vi "MEMR.vi"(11 "Expt State":T6) -> ()   [LabVIEW 2020]
uses:
  CFTS Main Panel SubVIs/CFTS-Experiment State.ctl
  Typedefs/MEMR-Sequence Step.ctl
panel:
  in  "Run":i32
  in  "Number":i32
  in  "ID":string
  out "exit signal":bool
  in  "Sampling rate (Hz)":dbl
  in  "Save raw data?":bool
  in  "Analysis":T1
  in  "Repeats":i32
  in  "Timing":T2
  in  "Sequence":T3
  in  "Elicitor":T4
  in  "Probe":T5
  out "Cal files":string
  out "show cal names":bool
  in  "file pattern":path
  in  "Start":bool
  in  "Stop":bool
  out "running":bool
  out "analysis":errorcluster
  out "finished":errorcluster
  out "restore defaults":bool
  out "ProgressBar":u8(slide) caption="Slide" scale=0.0..28.0
  out "FreqGraph":cluster{dbl[], dbl[]}(graph)
  out "IOGraph":cluster{dbl[], dbl[]}[](graph)
  out "TimeGraph":dbl[][](graph)
  out "GainSpectra":cluster{dbl[], dbl[]}[](graph)
  # "Probe"
  # "Elicitor"
  # "Timing"
  # "Analysis"
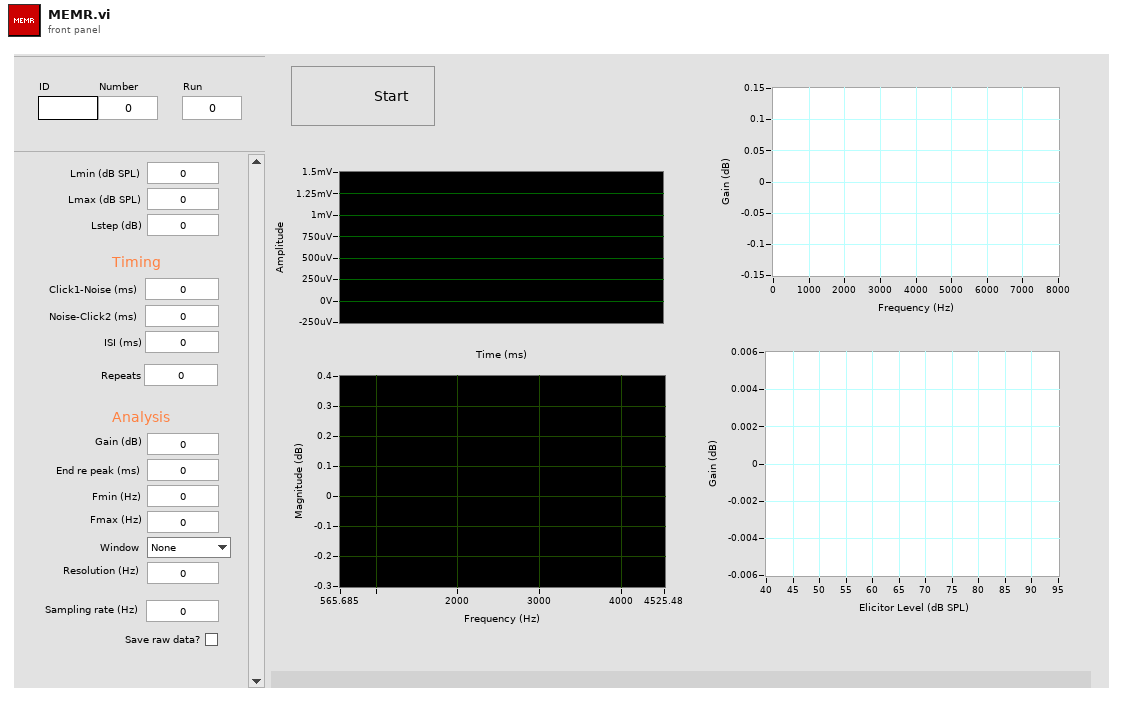
[diagram p1: front panel]
types:
  T1 = cluster{"T(ms) re peak":dbl, "Fmin (Hz)":dbl, "Fmax (Hz)":dbl, "Window":enum16{"None", "Hanning", "Hamming"}, "Gain (dB)":dbl, "Resol (Hz)":dbl}
  T2 = cluster{"Click1-Noise (ms)":dbl, "Noise-Click2 (ms)":dbl, "ISI (ms)":dbl}
  T3 = cluster{"Lmin (dB SPL)":dbl, "Lmax (dB SPL)":dbl, "Lstep (dB)":dbl}
  T4 = cluster{"Duration (ms)":dbl, "Ramp (ms)":dbl, "Transducer":enum16{"Insert", "TDH-39", "HD300", "ER-10X"}}
  T5 = cluster{"Ear":enum16{"Right", "Left"}, "Stimulus":enum16{"Click", "Chirp"}, "Duration (us)":dbl, "Level (dB pSPL)":dbl}
  T6 = typedef "CFTS-Experiment State.ctl" = cluster{"Experimenter":string, "Number":u32, "Right":string, "Left":string, "Data Folder":path, "State File":path, "Version Info":string, "End Exposure Time":dbl, "Exposure Duration":string, "Run #":cluster{"CAP":i16, "ABR":i16, "DP":i16, "VsEP":i16, "MeasSeq":i16, "SubSeq":i16, "SFOAE":i16}}
  T7 = typedef "MEMR-IPC.ctl" = cluster{"SGDA":refnum<queue>, "AnalysisStart":refnum<queue>, "AnalysisUpdate":refnum<queue>}
  T8 = cluster{"Run":refnum<vi>, "ProgressBar":refnum<vi>, "IOGraph":refnum<vi>, "TimeGraph":refnum<vi>, "FreqGraph":refnum<vi>, "GainSpectra":refnum<vi>}
  T9 = typedef "MEMR-Params.ctl" = cluster{"Probe":T10, "Elicitor":T11, "Sequence":T13, "Analysis":T14, "Repeats":i32, "Timing":T15, "Save raw":bool, "Fs (Hz)":dbl}
  T10 = typedef "MEMR-Probe.ctl" = cluster{"Ear":enum16{"Right", "Left"}, "Stimulus":enum16{"Click", "Chirp"}, "Duration (us)":dbl, "Level":dbl}
  T11 = typedef "MEMR-Elicitor.ctl" = cluster{"Duration (ms)":dbl, "Ramp (ms)":dbl, "Transducer":T12}
  T12 = typedef "HSTS-Transducer.ctl" = enum16{"Insert", "TDH-39", "HD300", "ER-10X"}
  T13 = typedef "MEMR-Sequence.ctl" = cluster{"Start":dbl, "Stop":dbl, "Step":dbl}
  T14 = typedef "MEMR-Analysis.ctl" = cluster{"T(ms) re peak":dbl, "Fmin (Hz)":dbl, "Fmax (Hz)":dbl, "Window":enum16{"None", "Hanning", "Hamming"}, "Gain (dB)":dbl, "Resol (Hz)":dbl}
  T15 = typedef "MEMR-Timing.ctl" = cluster{"Click1-Noise (ms)":dbl, "Noise-Click2 (ms)":dbl, "ISI (ms)":dbl}
  T16 = typedef "MEMR-Sequence Step.ctl" = cluster{"seq":i32, "rep":i32}
  T17 = typedef "MEMR-AO Data.ctl" = cluster{"Pulses":dbl[], "noiseChan":T18, "Fs (Hz)":dbl, "Npts":i32, "mults":dbl[], "chans":i32[], "Nreps":i32}
  T18 = typedef "Stimulus Channel (G3).xctl/Full Stimulus Channel Data.ctl" = cluster{"Waveform":T19, "Filter":T38, "Burst":T41, "Level":T42, "Name":string, "Advanced":T44, "SAM":T45, "Destination":T46}
  T19 = typedef "Waveform (G3).xctl/Waveform Data.ctl" = cluster{"Type":T20, "Tone":T21, "Pulse Train":T22, "Noise":T25, "File":T28, "FMSweep":T29, "Chirp Train":T30, "Complex Tone":cluster{"Params":T32, "Data":T34}, "FM":T35, "Vowel":T36, "Ramp":T37}
  T20 = typedef "Waveform Enum (V3).ctl" = enum16{"OFF", "Tone", "Noise", "Pulse Train", "File", "FM Sweep", "Chirp Train", "Complex Tone", "FM Tone", "Vowel", "Ramp"}
  T21 = typedef "Tone (G3).xctl/Tone.Properties.ctl" = cluster{"Frequency (kHz)":dbl, "Phase (cycles)":dbl, "Random phase":bool}
  T22 = typedef "Pulse Train Params.ctl" = cluster{"Pulse width (us)":dbl, "Pulse rate (Hz)":dbl, "Gap (ms)":dbl, "Polarity":T23, "PT State":T24, "Asynch":bool}
  T23 = typedef "Pulse Polarity.ctl" = enum16{"POS", "NEG", "POS-NEG", "NEG-POS"}
  T24 = typedef "PT-Continuous State.ctl" = cluster{"Template":dbl[], "Nperiod":i32, "Index":i32, "Pulse Rate (Hz)":dbl, "Phase (cycles)":dbl, "Noff":i32}
  T25 = typedef "Noise (G3).ctl" = cluster{"Properties":T26, "Data":T27}
  T26 = typedef "Noise (G3).Properties.ctl" = cluster{"InvFilt":bool, "Aweight":bool, "Seed":i32, "Tokens":i32, "Brickwall":bool}
  T27 = typedef "Noise (G3).Data.ctl" = cluster{"TokenNum":i32}
  T28 = typedef "StimFile-Params.ctl" = cluster{"Filename":path, "Signal":dbl[], "Channel":i32, "stream":bool, "offset":i32, "nreps":i32, "loops":i32, "Randomize":bool, "order":i32[], "Seed":i32, "Tokens":i32}
  T29 = typedef "FM Sweep Params.ctl" = cluster{"Rate (oct/s)":dbl, "Fmin (Hz)":dbl, "Fmax (Hz)":dbl, "Ramp (ms)":dbl, "Linear":bool}
  T30 = typedef "Chirp Train.ctl" = cluster{"Params":T31, "Data":cluster{"WF":dbl[]}}
  T31 = typedef "Chirp Train Params.ctl" = cluster{"Fmin (kHz)":dbl, "Fmax (kHz)":dbl, "Compensate":bool, "Duration (ms)":dbl}
  T32 = typedef "CT-Params.ctl" = cluster{"F0 (Hz)":dbl, "Band":cluster{"Flow (Hz)":dbl, "Fhigh (Hz)":dbl}, "Phase":T33, "Min F0 (Hz)":dbl, "Max F0 (Hz)":dbl, "ContinRandPhase":bool, "Max peak factor":dbl, "Max mod depth":dbl, "MinHarmNum":i32, "MaxHarmNum":i32, "Level Mode":enum16{"per component", "overall rms"}, "% jitter":dbl}
  T33 = typedef "CT-Phase Enum.ctl" = enum16{"Cosine", "Random", "Alternating"}
  T34 = typedef "CT-Runtime Data.ctl" = cluster{"Ncomp":i32, "MinHarm":i32, "Phase":dbl[], "Amplitude":dbl[], "Npts/frame":i32, "Last F0":dbl, "Fmin":dbl, "Fmax":dbl, "Lslope":dbl, "randphase":bool, "overall rms":bool, "fmult":dbl[], "jittered":bool}
  T35 = typedef "FM Tone.xctl/Data.ctl" = cluster{"Carrier (kHz)":dbl, "ModRate (Hz)":dbl, "Depth (Hz)":dbl, "Phase (cycles)":dbl}
  T36 = typedef "Vowel.xctl/Vowel.Properties.ctl" = cluster{"Freqs":string, "Set level":enum16{"Total", "Per component"}, "Freq":dbl[], "weights":dbl[]}
  T37 = typedef "Ramp.Properties.ctl" = cluster{"Duration (ms)":dbl}
  T38 = typedef "Filter (G3).xctl/Filter Data.ctl" = cluster{"Type":T39, "CF (kHz)":dbl, "BW (kHz)":dbl, "Cascade":bool, "Quadrature":bool, "Scale Factor":dbl, "Stages":cluster{"IIR Filter":cluster{"filter structure":enum32{"IIR 2nd Order", "IIR 4th Order"}, "Reverse Coefficients":dbl[], "Forward Coefficients":dbl[]}, "State":dbl[]}[], "Class":enum16{"Elliptic", "Butterworth"}, "Order":i32, "BWUnits":T40}
  T39 = typedef "Filter (G3).xctl/Filter Type.ctl" = enum16{"OFF", "Lowpass", "Highpass", "Bandpass", "Bandstop"}
  T40 = typedef "Filter-Bandwidth Units.ctl" = enum16{"Linear", "Octaves", "Min-Max"}
  T41 = typedef "Burst Control.xctl/Burst Data.ctl" = cluster{"Active":bool, "Delay (ms)":dbl, "Duration (ms)":dbl, "Ramp (ms)":dbl, "Rate (Hz)":dbl, "Trepeat (ms)":dbl, "Repeat":bool}
  T42 = typedef "Level (G3).xctl/Level Data.ctl" = cluster{"Level":dbl, "Units":T43, "Max":dbl, "Data":cluster{"Multiplier":dbl, "Cal File":path, "Cal":cluster{"Freq (Hz)":dbl[], "Mag (dB SPL)":dbl[], "Phase (deg)":dbl[]}, "audiogram":path}}
  T43 = typedef "Level (G3).xctl/Level Units (G3).ctl" = enum16{"dB atten", "dB SPL", "dB re 1 Vrms", "dB V/Hz½", "mW", "dB HL", "Volts", "dB mW"}
  T44 = typedef "Advanced Options (G3).xctl/Advanced Options (G3).ctl" = cluster{"AltPol":bool, "Var":string, "Expr":string}
  T45 = typedef "SAM Params.ctl" = cluster{"Active":bool, "Frequency (Hz)":dbl, "Depth":dbl, "Init Phase (cycles)":dbl, "phase (degrees)":dbl, "Asynch":bool}
  T46 = typedef "Destination.ctl" = cluster{"Name":string, "Num":i32}
  T47 = cluster{bool, "AI Waveforms":dbl[][], "Step In":T16}
  T48 = typedef "MEMR-Analysis State.ctl" = cluster{"Data file":path, "Raw":refnum<file>, "PT":cluster{"Freq":dbl[], "Mag":dbl[]}, "IO":cluster{"Level":dbl[], "Mag":dbl[], "NF":dbl[]}, "Nreps":i32, "Fs (Hz)":dbl, "Sum":dbl[], "Nplot":i32, "Noff":i32, "Gain":dbl, "spectra":cluster{"Freq":dbl[], "Mag":dbl[][]}[], "gain":cluster{"Freq":dbl[], "Mag":dbl[]}[], "Baseline":dbl[]}
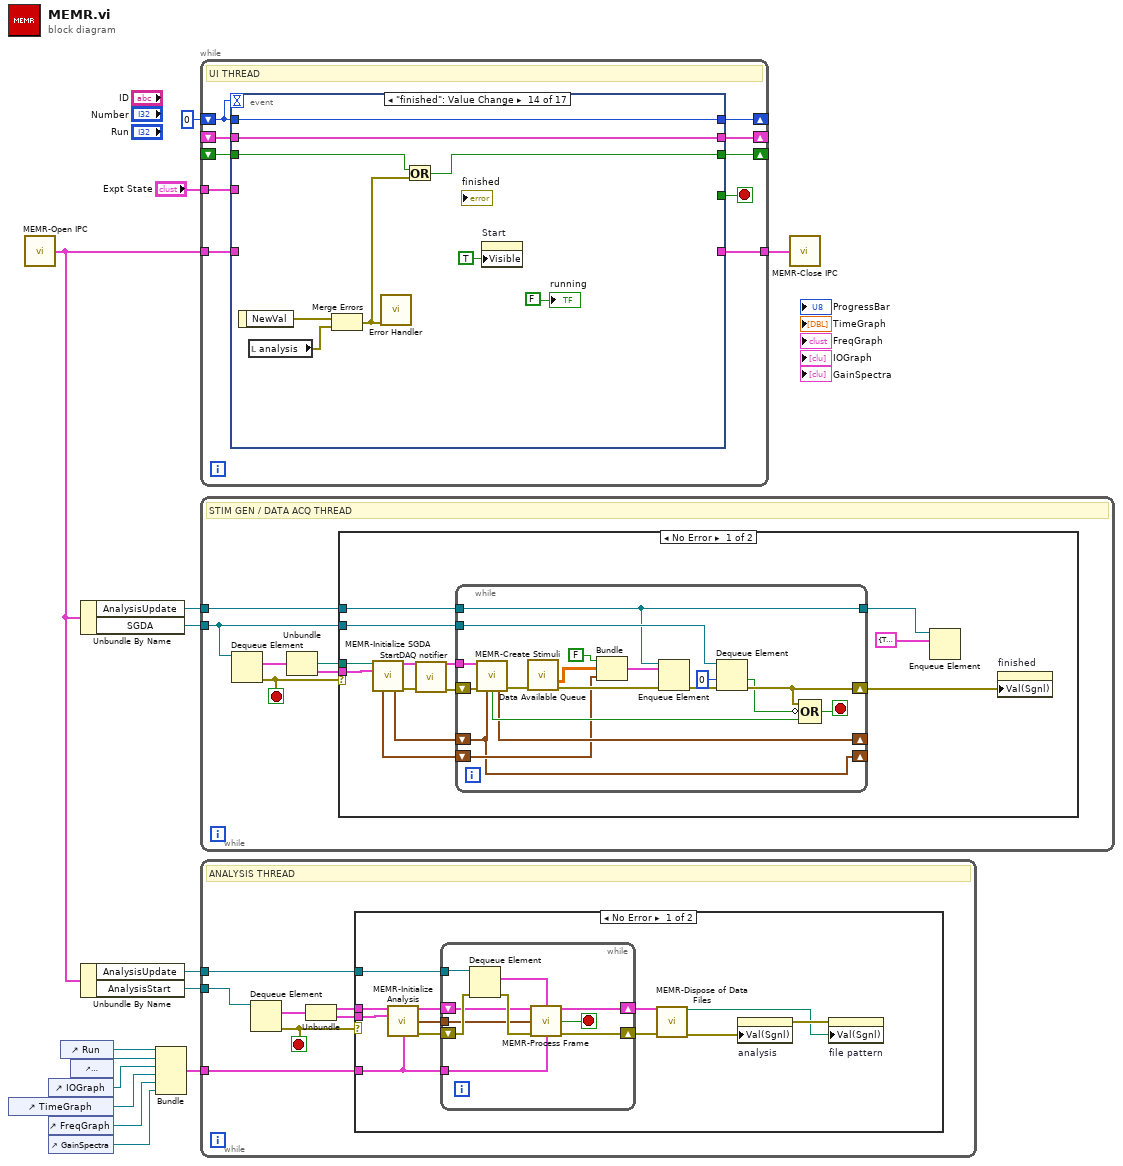
[diagram p0: block diagram]
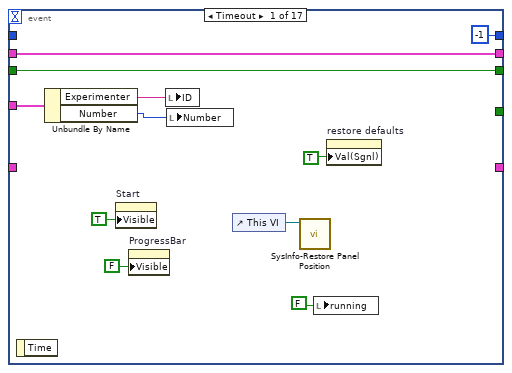
[diagram p3: hidden frame]
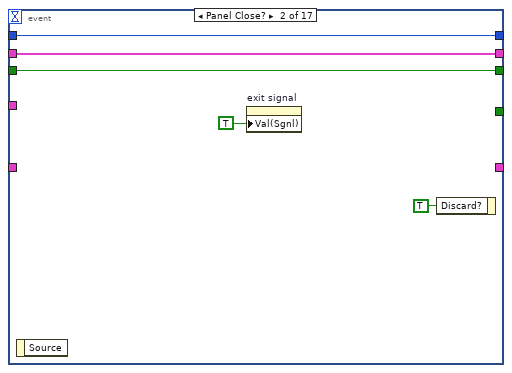
[diagram p4: hidden frame]
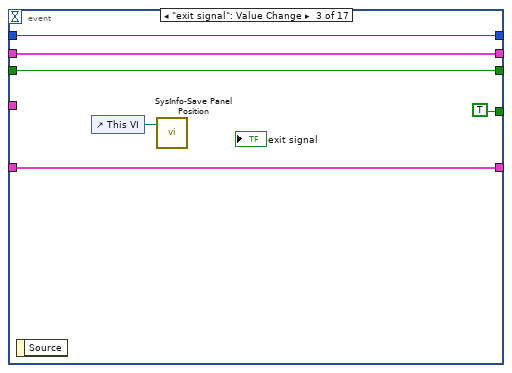
[diagram p5: hidden frame]
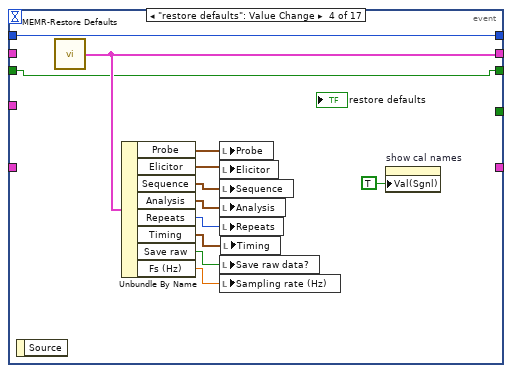
[diagram p6: hidden frame]
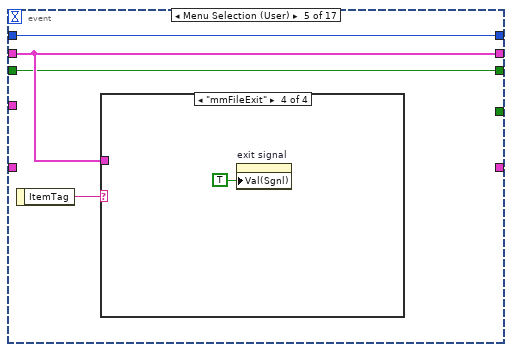
[diagram p7: hidden frame]
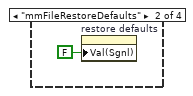
[diagram p9: hidden frame]
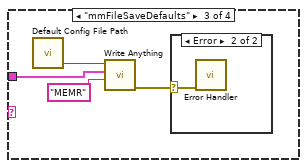
[diagram p10: hidden frame]
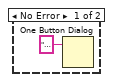
[diagram p11: hidden frame]
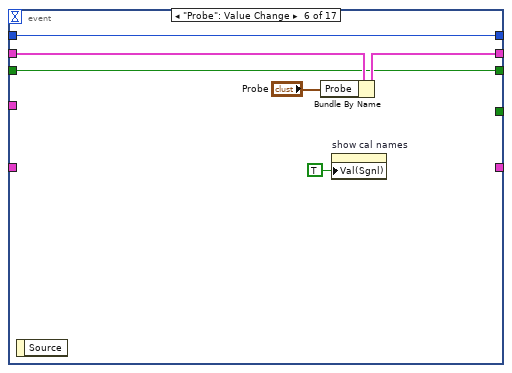
[diagram p12: hidden frame]
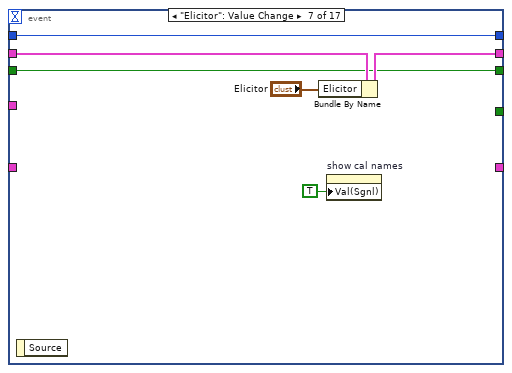
[diagram p13: hidden frame]
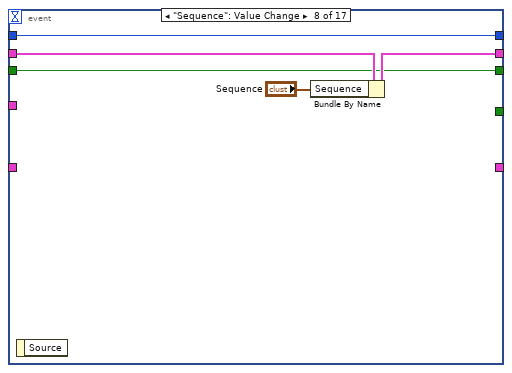
[diagram p14: hidden frame]
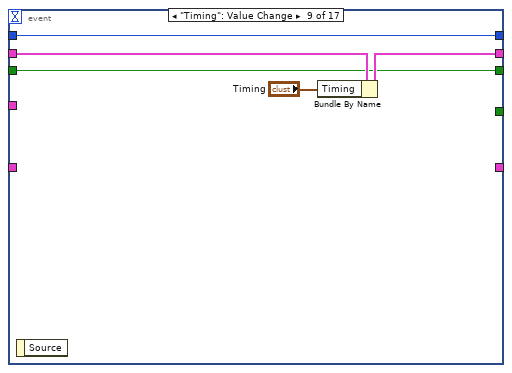
[diagram p15: hidden frame]
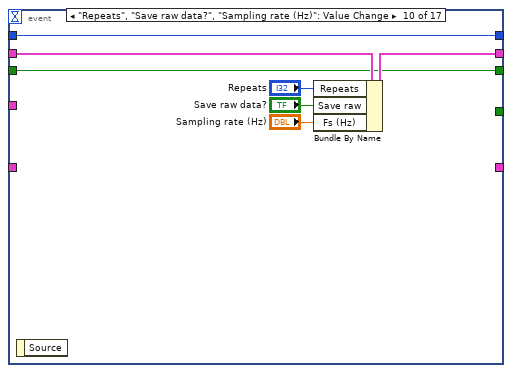
[diagram p16: hidden frame]
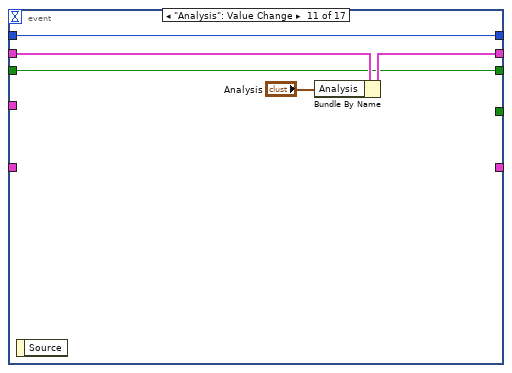
[diagram p17: hidden frame]
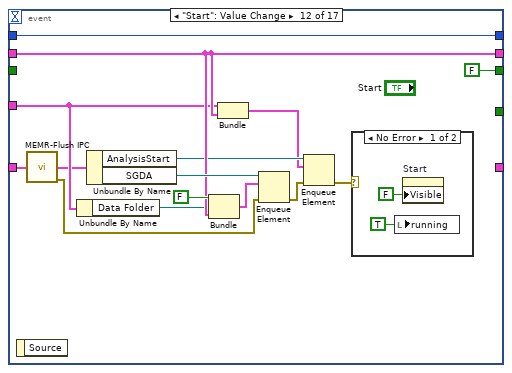
[diagram p18: hidden frame]
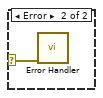
[diagram p19: hidden frame]
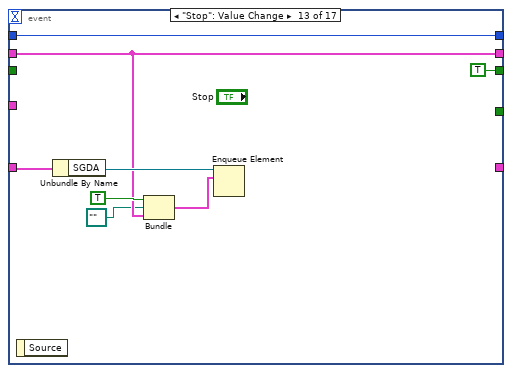
[diagram p20: hidden frame]
diagram:
  n1 = control-ref of="TimeGraph"() -> (w5:refnum<vi>)
  n2 = call "MEMR-Open IPC.vi"() -> ("IPC"=w13:T7)  [unwired: 15 in]
  n3 = control-ref of="IOGraph"() -> (w2:refnum<vi>)
  n4 = control-ref of="FreqGraph"() -> (w4:refnum<vi>)
  n5 = control-ref of="GainSpectra"() -> (w1:refnum<vi>)
  n6 = control-ref of="Run"() -> (w7:refnum<vi>)
  n7 = control-ref of="ProgressBar"() -> (w6:refnum<vi>)
  n8 = Unbundle By Name(w13) -> ("AnalysisUpdate"=w9:refnum<queue>, "SGDA"=w12:refnum<queue>)
  n9 = Unbundle By Name(w13) -> ("AnalysisUpdate"=w8:refnum<queue>, "AnalysisStart"=w11:refnum<queue>)
  n10 = Bundle("Run"=w7, "ProgressBar"=w6, "IOGraph"=w2, "TimeGraph"=w5, "FreqGraph"=w4, "GainSpectra"=w1) -> (w3:T8)  [unwired: 1 in]
  n11 = while {
    shift-right: [w24] -> _
    shift-left: 0 -> [w25]
    shift-right: [w22] -> _
    shift-left: _ -> [w21]
    tunnel: "Expt State" -> [w20]
    tunnel: w13 -> [w19]
    tunnel: [w18] -> w10
    shift-right: [w17] -> _
    shift-left: _ -> [w16]
    stop <- w23 stop-if-true
    # "UI THREAD"
    n12 = event shown="[13] \"finished\": Value Change" {
      selector: _ -> [_ _ _ _ _ _ _ _ _ _ _ _ _ _ _ _ _]
      dyn-events: _ -> [_ _ _ _ _ _ _ _ _ _ _ _ _ _ _ _ _]
      timeout: w25 -> [_ _ _ _ _ _ _ _ _ _ _ _ _ _ _ _ _]
      tunnel: w25 -> [_ w41 w47 w59 w63 w77 w83 w88 w93 w100 w105 w120 w131 w140 w148 w159 w184]
      tunnel: [-1 w41 w47 w59 w63 w77 w83 w88 w93 w100 w105 w120 w131 w140 w148 w159 w184] -> w24
      tunnel: [_ _ TRUE _ _ _ _ _ _ _ _ _ _ _ _ _ _] -> w23
      tunnel: [w34 w38 w45 w58 w61 w75 w81 w86 w91 w98 w103 w116 w126 w139 w144 w158 w175] -> w22
      tunnel: w21 -> [w34 w38 w45 _ w61 w76 w82 w87 w92 w99 w104 w116 w126 w139 w144 w158 w175]
      tunnel: w20 -> [w32 _ _ _ _ _ _ _ _ _ _ w111 _ _ _ _ w182]
      tunnel: w19 -> [_ _ w43 _ _ _ _ _ _ _ _ w109 w130 _ w146 _ _]
      tunnel: [_ _ w43 _ _ _ _ _ _ _ _ _ _ _ _ _ _] -> w18
      tunnel: [w26 w37 w42 w49 w60 w73 w79 w84 w89 w94 w101 FALSE ("file query") TRUE w132 w142 w156 w183] -> w17
      tunnel: w16 -> [w26 w37 w42 w49 w60 w73 w79 w84 w89 w94 w101 _ _ w133 w142 w156 w183]
      event Timeout {
        n13 = event-data() -> ()  [unwired: 1 in, 1 out]
        n14 = Unbundle By Name(w32) -> ("Experimenter"=w31:string, "Number"=w30:u32)
        n15 = property on="Start" class="Bool"("Visible"=TRUE) -> ()  [unwired: 2 in, 2 out]
        n16 = property on="ProgressBar" class="Slide (strict)"("Visible"=FALSE) -> ()  [unwired: 2 in, 2 out]
        n17 = local write "ID"(w31) -> ()
        n18 = local write "Number"(w30) -> ()
        n19 = control-ref of="This VI"() -> (w33:refnum<vi>)
        n20 = call "SysInfo-Restore Panel Position.vi"("VI Refnum"=w33) -> ()  [unwired: 12 in, 3 out]
        n21 = local write "running"(FALSE ("running")) -> ()
        n22 = property on="restore defaults" class="Bool (strict)"("Val(Sgnl)"=TRUE ("Value (Signaling)")) -> ()  [unwired: 2 in, 2 out]
      }
      event Panel Close? {
        n23 = event-data() -> ()  [unwired: 1 in, 1 out]
        n24 = property on="exit signal" class="Bool (strict)"("Val(Sgnl)"=TRUE ("Value (Signaling)")) -> ()  [unwired: 2 in, 2 out]
        n25 = event-data("Discard?"=TRUE) -> ()  [unwired: 1 in, 1 out]
      }
      event "exit signal": Value Change {
        n26 = event-data() -> ()  [unwired: 1 in, 1 out]
        n27 = control-ref of="This VI"() -> (w44:refnum<vi>)
        n28 = call "SysInfo-Save Panel Position.vi"("VI Refnum"=w44) -> ()  [unwired: 14 in, 1 out]
      }
      event "restore defaults": Value Change {
        n29 = event-data() -> ()  [unwired: 1 in, 1 out]
        n30 = call "MEMR-Restore Defaults.vi"() -> ("Params"=w58:T9)  [unwired: 15 in]
        n31 = Unbundle By Name(w58) -> ("Probe"=w57:T10, "Elicitor"=w56:T11, "Sequence"=w55:T13, "Analysis"=w54:T14, "Repeats"=w53:i32, "Timing"=w52:T15, "Save raw"=w51:bool, "Fs (Hz)"=w50:dbl)
        n32 = local write "Probe"(w57) -> ()
        n33 = local write "Elicitor"(w56) -> ()
        n34 = local write "Sequence"(w55) -> ()
        n35 = local write "Analysis"(w54) -> ()
        n36 = local write "Repeats"(w53) -> ()
        n37 = local write "Save raw data?"(w51) -> ()
        n38 = local write "Sampling rate (Hz)"(w50) -> ()
        n39 = local write "Timing"(w52) -> ()
        n40 = property on="show cal names" class="Bool (strict)"("Val(Sgnl)"=TRUE ("Value (Signaling)")) -> ()  [unwired: 2 in, 2 out]
      }
      event Menu Selection (User) {
        n41 = event-data() -> ("ItemTag"=w62:string)  [unwired: 1 in]
        n42 = case shown="\"mmFileExit\"" w62 {
          tunnel: w61 -> [_ _ w67 _]
          frame "False", Default {
          }
          frame "mmFileRestoreDefaults" {
            n43 = property on="restore defaults" class="Bool (strict)"("Val(Sgnl)"=FALSE ("Value (Signaling)")) -> ()  [unwired: 2 in, 2 out]
          }
          frame "mmFileSaveDefaults" {
            n44 = call "Default Config File Path.vi"() -> ("Default config file name"=w68:path)
            n45 = call "Write Anything.vi"("Section Name (Name of \"Anything\")"="MEMR" ("Section Name (Name of \"Anything\")"), "Anything"=w67, "Path (dialog)"=w68) -> ("Error Out"=w65:errorcluster)  [unwired: 7 in, 1 out]
            n46 = case shown="Error" w65 {
              selector: w65 -> [_ w70]
              frame No Error {
                n47 = One Button Dialog(message="Defaults saved.") -> ()  [unwired: 1 in, 1 out]
              }
              frame Error {
                n48 = call "Error Handler.vi"("error in (no error)"=w70) -> ()  [unwired: 13 in, 2 out]
              }
            }
          }
          frame "mmFileExit" {
            n49 = property on="exit signal" class="Bool (strict)"("Val(Sgnl)"=TRUE ("Value (Signaling)")) -> ()  [unwired: 2 in, 2 out]
          }
        }
      }
      event "Probe": Value Change {
        n50 = event-data() -> ()  [unwired: 1 in, 1 out]
        n51 = Bundle By Name(cluster=w76, "Probe"="Probe") -> (w75:T9)
        n52 = property on="show cal names" class="Bool (strict)"("Val(Sgnl)"=TRUE ("Value (Signaling)")) -> ()  [unwired: 2 in, 2 out]
      }
      event "Elicitor": Value Change {
        n53 = event-data() -> ()  [unwired: 1 in, 1 out]
        n54 = Bundle By Name(cluster=w82, "Elicitor"="Elicitor") -> (w81:T9)
        n55 = property on="show cal names" class="Bool (strict)"("Val(Sgnl)"=TRUE ("Value (Signaling)")) -> ()  [unwired: 2 in, 2 out]
      }
      event "Sequence": Value Change {
        n56 = event-data() -> ()  [unwired: 1 in, 1 out]
        n57 = Bundle By Name(cluster=w87, "Sequence"="Sequence") -> (w86:T9)
      }
      event "Timing": Value Change {
        n58 = event-data() -> ()  [unwired: 1 in, 1 out]
        n59 = Bundle By Name(cluster=w92, "Timing"="Timing") -> (w91:T9)
      }
      event "Repeats", "Save raw data?", "Sampling rate (Hz)": Value Change {
        n60 = event-data() -> ()  [unwired: 1 in, 1 out]
        n61 = Bundle By Name(cluster=w99, "Repeats"="Repeats", "Save raw"="Save raw data?", "Fs (Hz)"="Sampling rate (Hz)") -> (w98:T9)
      }
      event "Analysis": Value Change {
        n62 = event-data() -> ()  [unwired: 1 in, 1 out]
        n63 = Bundle By Name(cluster=w104, "Analysis"="Analysis") -> (w103:T9)
      }
      event "Start": Value Change {
        n64 = event-data() -> ()  [unwired: 1 in, 1 out]
        n65 = call "MEMR-Flush IPC.vi"("IPC"=w109) -> ("IPC thru"=w108:T7, "error out"=w107:errorcluster)  [unwired: 13 in]
        n66 = Unbundle By Name(w111) -> ("Data Folder"=w110:path)
        n67 = Unbundle By Name(w108) -> ("AnalysisStart"=w115:refnum<queue>, "SGDA"=w119:refnum<queue>)
        n68 = Bundle(FALSE, "Data Folder"=w110, "Params"=w116) -> (w117:cluster{bool, "Data Folder":path, "Params":T9})  [unwired: 1 in]
        n69 = Bundle("Expt State"=w111, "Params"=w116) -> (w114:cluster{"Expt State":T6, "Params":T9})  [unwired: 1 in]
        n70 = Enqueue Element(queue=w119, element=w117, error in (no error)=w107) -> (error out=w113:errorcluster)  [unwired: 1 in, 2 out]
        n71 = Enqueue Element(queue=w115, element=w114, error in (no error)=w113) -> (error out=w112:errorcluster)  [unwired: 1 in, 2 out]
        n72 = case shown="No Error" w112 {
          selector: w112 -> [_ w123]
          frame No Error {
            n73 = local write "running"(TRUE ("running")) -> ()
            n74 = property on="Start" class="Bool"("Visible"=FALSE) -> ()  [unwired: 2 in, 2 out]
          }
          frame Error {
            n75 = call "Error Handler.vi"("error in (no error)"=w123) -> ()  [unwired: 13 in, 2 out]
          }
        }
      }
      event "Stop": Value Change {
        n76 = event-data() -> ()  [unwired: 1 in, 1 out]
        n77 = Unbundle By Name(w130) -> ("SGDA"=w128:refnum<queue>)
        n78 = Bundle(TRUE, path "", "Params"=w126) -> (w127:cluster{bool, path, "Params":T9})  [unwired: 1 in]
        n79 = Enqueue Element(queue=w128, element=w127) -> ()  [unwired: 2 in, 3 out]
      }
      event "finished": Value Change {
        n80 = event-data() -> ("NewVal"=w136:errorcluster)  [unwired: 1 in]
        n81 = local read "analysis"() -> (w135:errorcluster)
        n82 = Merge Errors(w136, w135) -> (w134:errorcluster)
        n83 = call "Error Handler.vi"("error in (no error)"=w134) -> ()  [unwired: 13 in, 2 out]
        n84 = Or(x=w133, y=w134) -> (x .or. y?=w132:bool)
        n85 = property on="Start" class="Bool"("Visible"=TRUE) -> ()  [unwired: 2 in, 2 out]
        "running" <- FALSE ("running")
      }
      event "analysis": Value Change {
        n86 = event-data() -> ("NewVal"=w143:errorcluster)  [unwired: 1 in]
        n87 = local read "running"() -> (w147:bool)
        n88 = Unbundle By Name(w146) -> ("SGDA"=w145:refnum<queue>)
        n89 = case shown="True" w147 {
          tunnel: w145 -> [_ w154]
          tunnel: w144 -> [_ w153]
          tunnel: w143 -> [w149 _]
          frame False {
            n90 = call "Error Handler.vi"("error in (no error)"=w149) -> ()  [unwired: 13 in, 2 out]
          }
          frame True {
            n91 = Bundle(TRUE, path "", "Params"=w153) -> (w150:cluster{bool, path, "Params":T9})  [unwired: 1 in]
            n92 = Enqueue Element(queue=w154, element=w150) -> ()  [unwired: 2 in, 3 out]
          }
        }
        n93 = property on="ProgressBar" class="Slide (strict)"("Visible"=FALSE) -> ()  [unwired: 2 in, 2 out]
      }
      event "file pattern": Value Change {
        n94 = event-data() -> ()  [unwired: 1 in, 1 out]
        n95 = case shown="True" w156 {
          tunnel: [TRUE ("T button?") w161] -> w155
          frame False {
          }
          frame True {
            n96 = Two Button Dialog(message="Data collection aborted.\nSave last file?", 1:"No" ("F button name (\"Cancel\")"), 2:"Yes" ("T button name (\"OK\")")) -> (T button?=w161:bool)
          }
        }
        n97 = case shown="False" w155 {
          tunnel: "file pattern" -> [w169 _]
          frame False {
            n98 = Strip Path(path=w169) -> (stripped path=w168:path, name=w167:string)
            n99 = List Folder(path=w168, pattern=w167) -> (path out=w166:path, filenames=w165:string[])  [unwired: 2 in, 2 out]
            n100 = for {
              tunnel: w166 -> [w173]
              tunnel: w165 -> [w172] mode=indexing
              tunnel: [w170] -> _
              n101 = Build Path(base path=w173, name or relative path=w172) -> (appended path=w171:path)
              n102 = Delete(path (use dialog)=w171) -> (error out=w170:errorcluster)  [unwired: 4 in, 2 out]
            }
          }
          frame True {
          }
        }
      }
      event "show cal names": Value Change {
        n103 = event-data() -> ()  [unwired: 1 in, 1 out]
        n104 = Unbundle By Name(w182) -> ("Data Folder"=w174:path)
        n105 = call "MEMR-Get Calibration Files.vi"("Params"=w175, "Data Folder"=w174) -> ("Probe"=w177:path, "Elicitor"=w176:path)  [unwired: 11 in, 1 out]
        n106 = Path To String(path=w177) -> (string=w180:string)
        n107 = Path To String(path=w176) -> (string=w179:string)
        n108 = property on="Ear" class="Enum (strict)"("TipStrip"=w180) -> ()  [unwired: 2 in, 2 out]
        n109 = Format Into String(format string="%s; %s", w180, w179) -> (resulting string=→"Cal files":string)  [unwired: 2 in, 1 out]
        n110 = property on="Transducer" class="Enum (strict)"("TipStrip"=w179) -> ()  [unwired: 2 in, 2 out]
      }
    }
  }
  n111 = while {
    tunnel: w12 -> [w185]
    tunnel: w9 -> [w186]
    stop <- w189 stop-if-true
    # "STIM GEN / DATA ACQ THREAD"
    n112 = Dequeue Element(queue=w185) -> (element=w190:cluster{bool, path, "Params":T9}, error out=w189:errorcluster)  [unwired: 2 in, 2 out]
    n113 = Unbundle(w190) -> (w188:path, "Params"=w187:T9)  [unwired: 1 out]
    n114 = case shown="No Error" w189 {
      tunnel: w188 -> [w202 _]
      tunnel: w187 -> [w201 _]
      tunnel: w186 -> [w197 _]
      tunnel: w185 -> [w195 _]
      frame No Error {
        n115 = call "MEMR-Initialize SGDA.vi"("Data folder"=w202, "Params"=w201) -> ("AO"=w200:T17, "Step In"=w191:T16, "Step Out"=w196:T16, "error out"=w199:errorcluster)  [unwired: 10 in]
        n116 = call "StartDAQ notifier.vi"("error in (no error)"=w199) -> ("error out"=w198:errorcluster)  [unwired: 6 in]
        n117 = while {
          tunnel: w200 -> [w220]
          tunnel: w197 -> [w207]
          shift-right: [w208] -> w192
          shift-left: w198 -> [w219]
          shift-right: [w213] -> _
          shift-left: w196 -> [w203]
          tunnel: w195 -> [w209]
          tunnel: [w207] -> w194
          shift-right: [w203] -> _
          shift-left: w191 -> [w204]
          stop <- w217 stop-if-true
          n118 = call "MEMR-Create Stimuli.vi"("AO"=w220, "error in (no error)"=w219, "Step In"=w203) -> ("finished"=w216:bool, "Step Out"=w213:T16, "error out"=w218:errorcluster)  [unwired: 10 in]
          n119 = call "Data Available Queue.vi"("error in (no error)"=w218) -> ("AI Waveforms"=w214:dbl[][], "error out"=w215:errorcluster)  [unwired: 10 in, 3 out]
          n120 = Bundle(FALSE, "AI Waveforms"=w214, "Step In"=w204) -> (w211:T47)  [unwired: 1 in]
          n121 = Enqueue Element(queue=w207, element=w211, error in (no error)=w215) -> (error out=w210:errorcluster)  [unwired: 1 in, 2 out]
          n122 = Dequeue Element(queue=w209, timeout in ms (-1)=0, error in (no error)=w210) -> (timed out?=w205:bool, error out=w208:errorcluster)  [unwired: 2 out]
          n123 = Compound Arithmetic op=OR(w208, invert w205, w216) -> (w217:bool)
        }
        n124 = Enqueue Element(queue=w194, element=cluster{bool, dbl[][], "Step Out":T16} {TRUE, [], "Step Out"={"seq"=0, "rep"=0}}) -> ()  [unwired: 2 in, 3 out]
        n125 = property on="finished" class="Clust (strict)"("Val(Sgnl)"=w192) -> ()  [unwired: 2 in, 2 out]
      }
      frame Error {
      }
    }
  }
  n126 = while {
    tunnel: w11 -> [w226]
    tunnel: w8 -> [w224]
    tunnel: w3 -> [w223]
    stop <- w225 stop-if-true
    # "ANALYSIS THREAD"
    n127 = Dequeue Element(queue=w226) -> (element=w227:cluster{"Expt State":T6, "Params":T9}, error out=w225:errorcluster)  [unwired: 2 in, 2 out]
    n128 = Unbundle(w227) -> ("Expt State"=w222:T6, "Params"=w221:T9)
    n129 = case shown="No Error" w225 {
      tunnel: w224 -> [w237 _]
      tunnel: w223 -> [w228 _]
      tunnel: w222 -> [w239 _]
      tunnel: w221 -> [w238 _]
      frame No Error {
        n130 = call "MEMR-Initialize Analysis.vi"("Expt State"=w239, "Params"=w238, "controls"=w228) -> ("State"=w236:T48, "Analysis"=w235:T14, "error out"=w234:errorcluster)  [unwired: 10 in]
        n131 = while {
          tunnel: w237 -> [w248]
          tunnel: w235 -> [w243]
          shift-right: [w246] -> w233
          shift-left: w234 -> [w249]
          shift-right: [w241] -> w232
          shift-left: w236 -> [w244]
          tunnel: w228 -> [w240]
          stop <- w242 stop-if-true
          n132 = Dequeue Element(queue=w248, error in (no error)=w249) -> (element=w245:cluster{bool, dbl[][], "Step Out":T16}, error out=w247:errorcluster)  [unwired: 1 in, 2 out]
          n133 = call "MEMR-Process Frame.vi"("State In"=w244, "queue data"=w245, "Analysis"=w243, "error in (no error)"=w247, "controls"=w240) -> ("State Out"=w241:T48, "finished"=w242:bool, "error out"=w246:errorcluster)  [unwired: 8 in]
        }
        n134 = call "MEMR-Dispose of Data Files.vi"("State"=w232, "error in (no error)"=w233) -> ("file pattern"=w229:path, "error out"=w231:errorcluster)  [unwired: 12 in]
        n135 = property on="analysis" class="Clust (strict)"("Val(Sgnl)"=w231) -> (error out=w230:errorcluster)  [unwired: 2 in, 1 out]
        n136 = property on="file pattern" class="Path"(error in=w230, "Val(Sgnl)"=w229) -> ()  [unwired: 1 in, 2 out]
      }
      frame Error {
      }
    }
  }
  n137 = call "MEMR-Close IPC.vi"("IPC"=w10) -> ()  [unwired: 15 in]
